vi "TestCMD.vi"(4 "QueueMotorCMD":refnum<queue>, 5 "ControlInterfce":variant, 6 "ID":string, 7 "MotorName":string) -> ()   [LabVIEW 2020]
panel:
  out "AddPath":T1(array[cluster])
  out "Speed":string
  out "Running?":bool=TRUE
  in  "CurrentPos":T2 {"X" format="%03.3f"; "Y" format="%3.3f"; "Z" format="%3.3f"; "U" format="%3.3f"; "V" format="%3.3f"; "W" format="%3.3f"; "H" format="%.3f"}
  out "CMD":T3
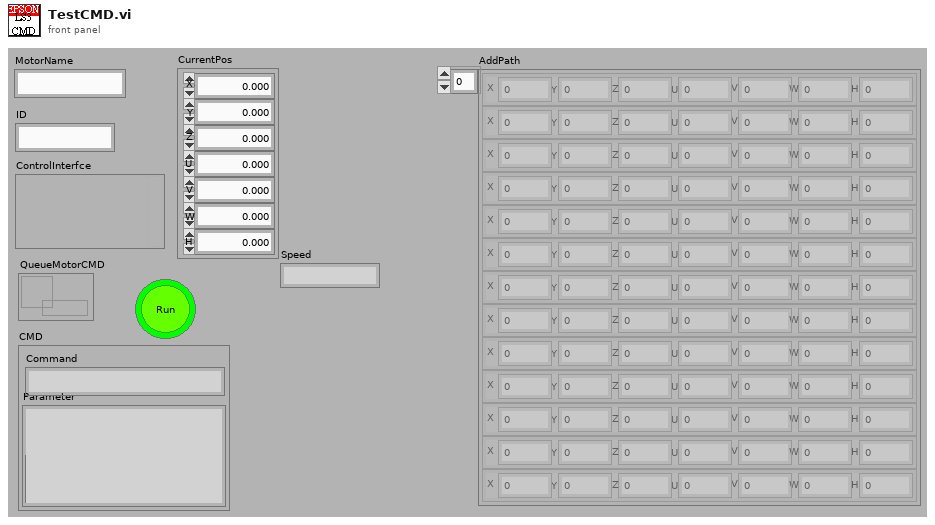
[diagram p1: front panel]
types:
  T1 = cluster{"X":sgl, "Y":sgl, "Z":sgl, "U":sgl, "V":sgl, "W":sgl, "H":sgl}[]
  T2 = cluster{"X":sgl, "Y":sgl, "Z":sgl, "U":sgl, "V":sgl, "W":sgl, "H":sgl}
  T3 = cluster{"Command":string, "Parameter":string, "queue out":refnum<queue>}
  T4 = enum16{"Get", "UpdatePointS", "Init", "UpdateIndex", "GetCurrent&Index+1", "GetWithIndex", "ChkLast"}
  T5 = enum16{"Get", "UpdatePointS", "Init", "UpdateIndex", "GetCurrent&Index+1", "GetWithIndex", "ChkLast", "GetCurrent"}
  T6 = cluster{cluster{"X":sgl, "Y":sgl, "Z":sgl, "U":sgl, "V":sgl, "W":sgl, "H":sgl}[]}
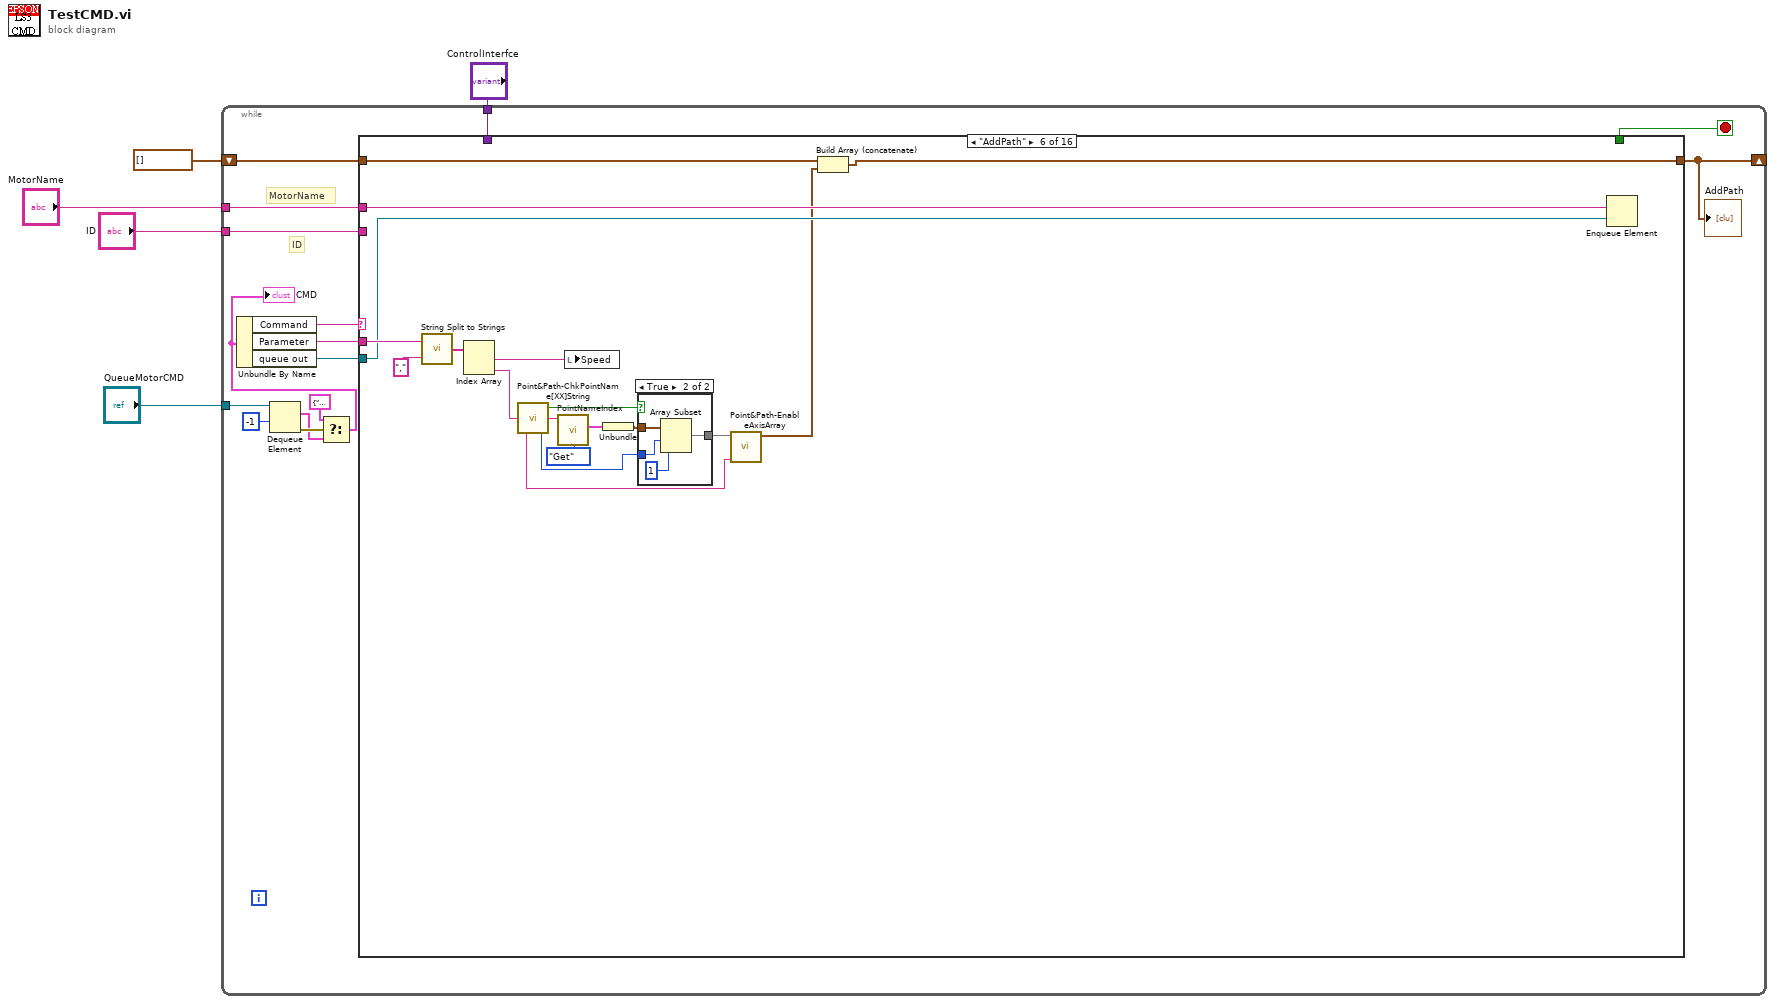
[diagram p0: block diagram]
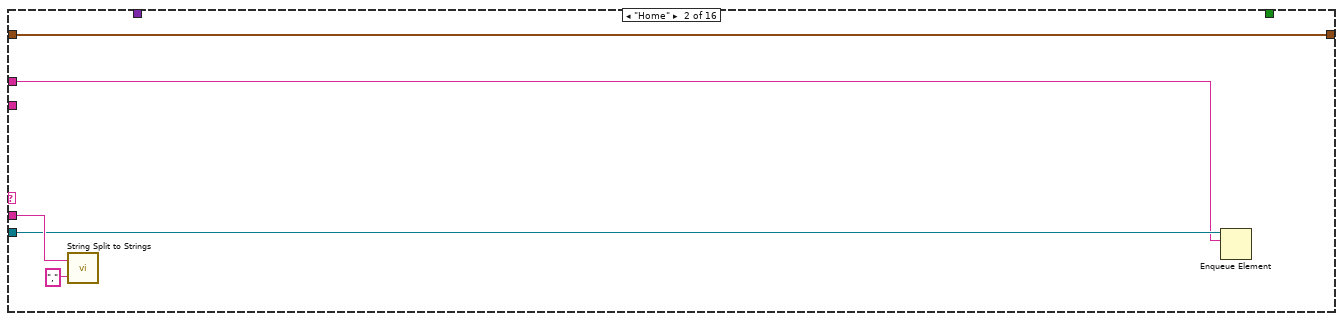
[diagram p3: hidden frame]
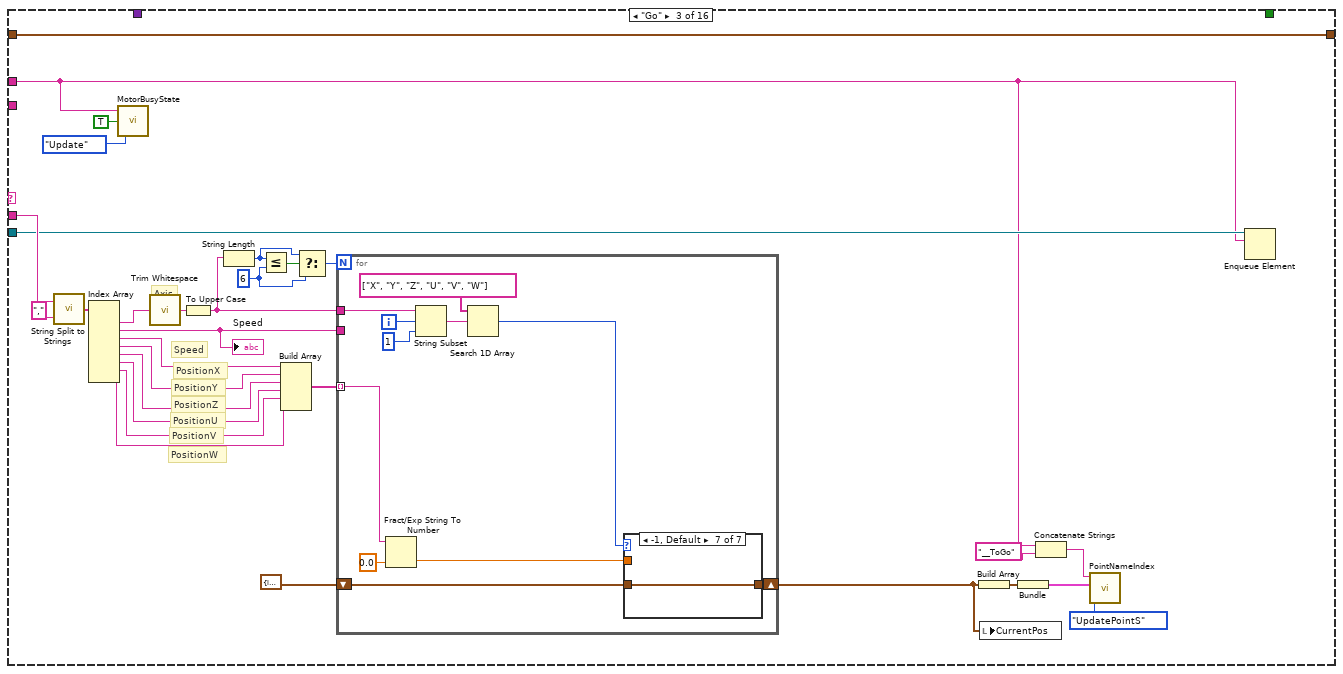
[diagram p4: hidden frame]
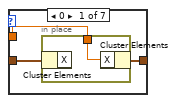
[diagram p5: hidden frame]
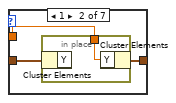
[diagram p6: hidden frame]
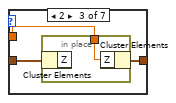
[diagram p7: hidden frame]
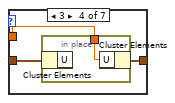
[diagram p8: hidden frame]
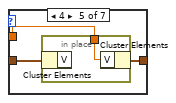
[diagram p9: hidden frame]
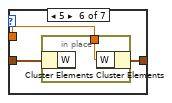
[diagram p10: hidden frame]
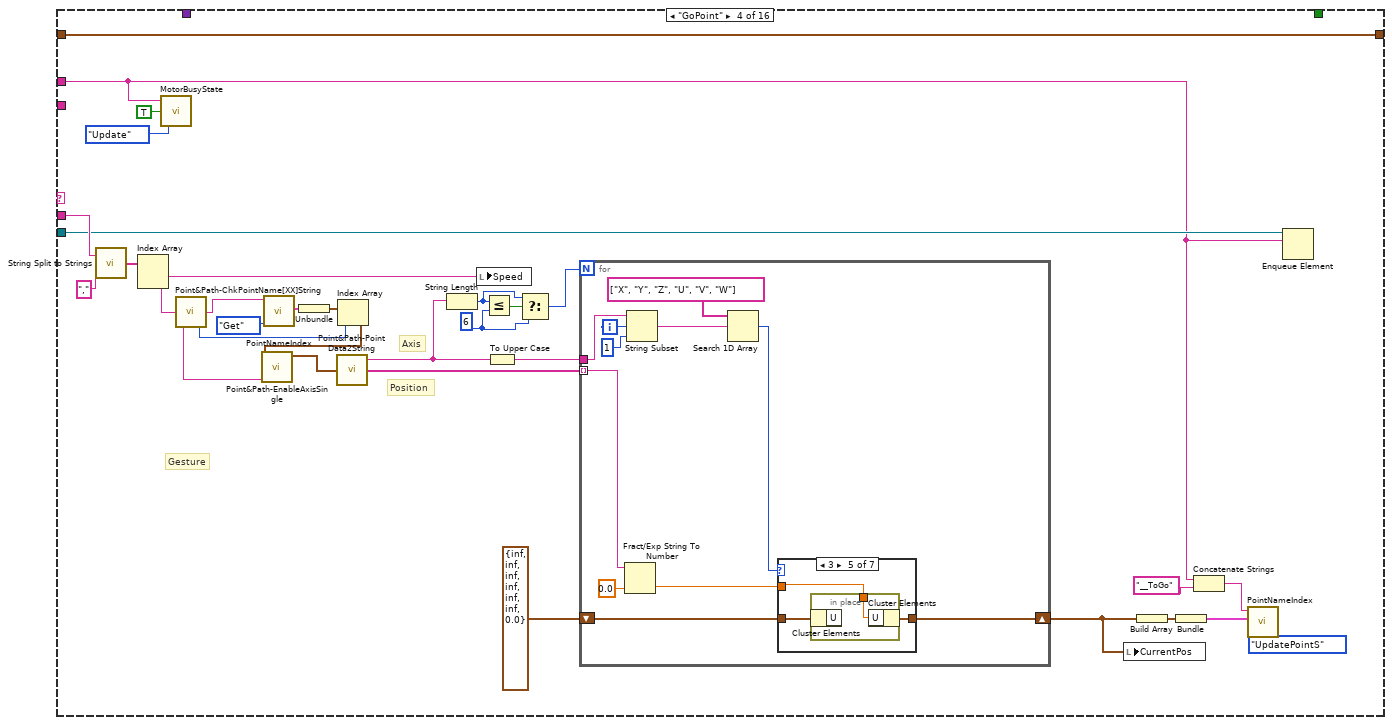
[diagram p11: hidden frame]
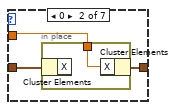
[diagram p13: hidden frame]
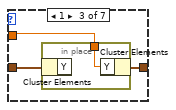
[diagram p14: hidden frame]
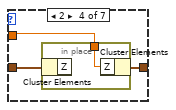
[diagram p15: hidden frame]
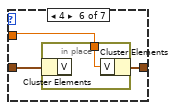
[diagram p16: hidden frame]
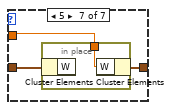
[diagram p17: hidden frame]
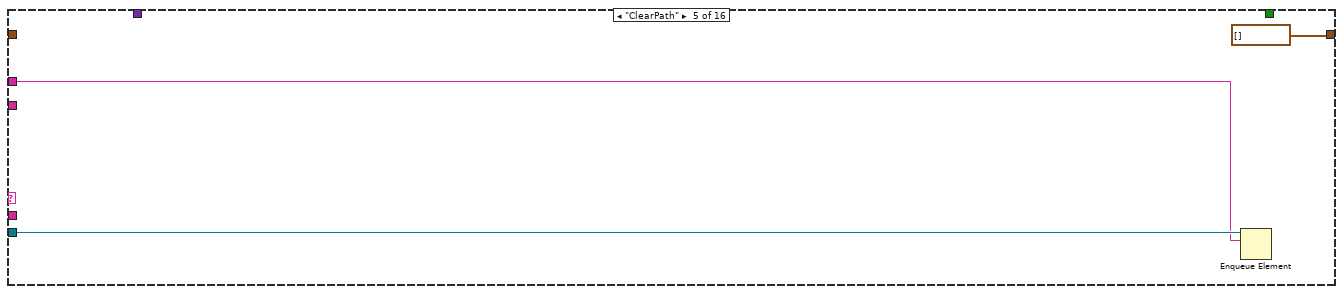
[diagram p18: hidden frame]
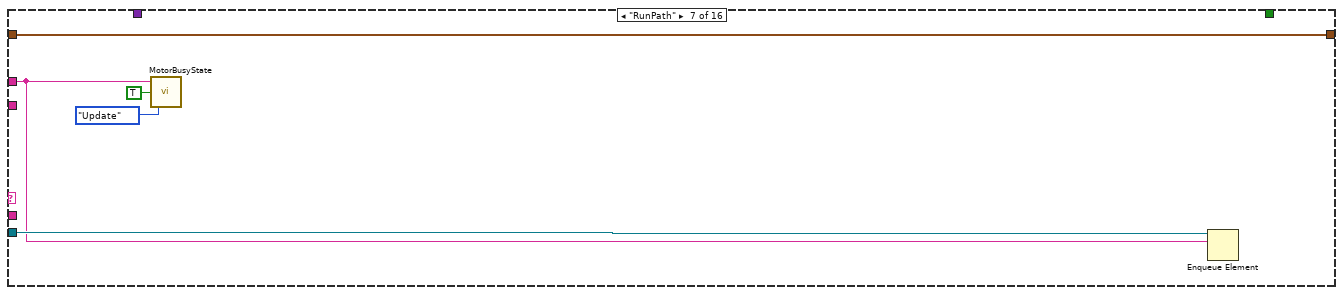
[diagram p20: hidden frame]
diagram:
  n1 = while {
    tunnel: "QueueMotorCMD" -> [w20]
    tunnel: "MotorName" -> [w16]
    tunnel: "ID" -> [w15]
    tunnel: "ControlInterfce" -> [w13]
    shift-right: [w6] -> _
    shift-left: T1 [] ("AddPath") -> [w7]
    stop <- w14 stop-if-true
    # "ID"
    # "MotorName"
    n2 = Dequeue Element(queue=w20, timeout in ms (-1)=-1) -> (element=w10:T3, error out=w11:errorcluster)  [unwired: 1 in, 2 out]
    n3 = Select(t=T3 {"Command"="Close", "Parameter"="", "queue out"=refnum} ("element"), s=w11, f=w10) -> (s? t:f=w9:T3)
    "CMD" <- w9
    n4 = Unbundle By Name(w9) -> ("Command"=w19:string, "Parameter"=w18:string, "queue out"=w17:refnum<queue>)
    n5 = case shown="\"AddPath\"" w19 {
      tunnel: w18 -> [_ w25 w48 w113 _ w176 _ _ _ _ _ _ _ _ _ _]
      tunnel: w17 -> [_ w24 w46 w106 w163 w170 w191 w194 w200 w205 w210 w214 _ w219 w223 _]
      tunnel: w16 -> [_ w23 w37 w99 w162 w174 w188 w193 w201 w207 w211 w213 _ _ _ _]
      tunnel: w15 -> [_ _ _ _ _ _ _ _ _ _ _ _ _ _ _ _]
      tunnel: [_ _ _ _ _ _ _ _ _ _ _ _ _ _ _ TRUE] -> w14
      tunnel: w13 -> [_ _ _ _ _ _ _ _ _ _ _ _ _ _ _ _]
      tunnel: w7 -> [w21 w22 w29 w93 _ w167 w187 w192 w195 w202 w209 w212 w215 w216 w220 w224]
      tunnel: [w21 w22 w29 w93 T1 [] ("AddPath") w166 w187 w192 w195 w202 w209 w212 w215 w216 w220 w224] -> w6
      frame "UpdateInfo", Default {
      }
      frame "Home" {
        n6 = call "String Split to Strings.vi"("search string/char (-)"=",", "String"=w25) -> ()  [unwired: 1 out]
        n7 = Enqueue Element(queue=w24, element=w23) -> ()  [unwired: 2 in, 3 out]
      }
      frame "Go" {
        w31 = 6 ("y")
        # "PositionW"
        # "PositionV"
        # "PositionU"
        # "PositionZ"
        # "PositionY"
        # "Speed"
        # "PositionX"
        # "Axis"
        n8 = call "String Split to Strings.vi"("search string/char (-)"=",", "String"=w48) -> ("Array"=w50:string[])
        n9 = Index Array(array=w50) -> (element #1=w51:string, element #2=w35:string, element #3=w52:string, element #4=w53:string, element #5=w54:string, element #6=w55:string, element #7=w28:string, element #8=w27:string)  [unwired: 8 in]
        "Speed" <- w35
        n10 = call "MotorBusyState.vi"("OP"=enum16{"Get", "Update", "Init"}."Update", "BusyStateIn"=TRUE, "MotorStateName"=w37) -> ()  [unwired: 1 in, 2 out]
        n11 = call <vilib>:"Trim Whitespace.vi"("string"=w51) -> ("trimmed string"=w56:string)  [unwired: 1 in]
        n12 = To Upper Case(1:w56) -> (0:w30:string)
        n13 = String Length(string=w30) -> (length=w33:i32)
        n14 = Less Or Equal?(x=w33, y=w31) -> (x <= y?=w34:bool)
        n15 = Build Array(w52, w53, w54, w55, w28, w27) -> (w47:string[])
        n16 = Select(t=w33, s=w34, f=w31) -> (s? t:f=w32:i32)
        n17 = for {
          N: w32 -> [_]
          tunnel: w30 -> [w64]
          tunnel: w47 -> [w61] mode=indexing
          shift-right: [w59] -> w36
          shift-left: T2 {"X"=inf, "Y"=inf, "Z"=inf, "U"=inf, "V"=inf, "W"=inf, "H"=0.0} ("PointData 2") -> [w62]
          tunnel: w35 -> [_]
          i -> [w65]
          n18 = Fract/Exp String To Number(string=w61, default (0 dbl)=sgl 0.0 ("default (0 DBL)")) -> (number=w57:sgl)  [unwired: 2 in, 1 out]
          n19 = String Subset(string=w64, offset (0)=w65, length (rest)=1 ("length (rest)")) -> (substring=w63:string)
          n20 = Search 1D Array(1D array=string[] ["X", "Y", "Z", "U", "V", "W"], element=w63) -> (index of element=w58:i32)  [unwired: 1 in]
          n21 = case shown="-1, Default" w58 {
            tunnel: w57 -> [w69 w73 w77 w81 w85 w89 _]
            tunnel: w62 -> [w70 w74 w78 w82 w86 w90 w92]
            tunnel: [w68 w72 w76 w80 w84 w88 w92] -> w59
            frame 0 {
              n22 = in-place {
                in-place-border: w69 -> [w71]
                n23 = in-place-cluster #1(w70) -> ()  [unwired: 1 out]
                n24 = in-place-cluster #1("X"=w71) -> (w68:T2)
              }
            }
            frame 1 {
              n25 = in-place {
                in-place-border: w73 -> [w75]
                n26 = in-place-cluster #2(w74) -> ()  [unwired: 1 out]
                n27 = in-place-cluster #2("Y"=w75) -> (w72:T2)
              }
            }
            frame 2 {
              n28 = in-place {
                in-place-border: w77 -> [w79]
                n29 = in-place-cluster #3(w78) -> ()  [unwired: 1 out]
                n30 = in-place-cluster #3("Z"=w79) -> (w76:T2)
              }
            }
            frame 3 {
              n31 = in-place {
                in-place-border: w81 -> [w83]
                n32 = in-place-cluster #4(w82) -> ()  [unwired: 1 out]
                n33 = in-place-cluster #4("U"=w83) -> (w80:T2)
              }
            }
            frame 4 {
              n34 = in-place {
                in-place-border: w85 -> [w87]
                n35 = in-place-cluster #5(w86) -> ()  [unwired: 1 out]
                n36 = in-place-cluster #5("V"=w87) -> (w84:T2)
              }
            }
            frame 5 {
              n37 = in-place {
                in-place-border: w89 -> [w91]
                n38 = in-place-cluster #6(w90) -> ()  [unwired: 1 out]
                n39 = in-place-cluster #6("W"=w91) -> (w88:T2)
              }
            }
            frame -1, Default {
            }
          }
        }
        n40 = Build Array(w36) -> (w43:T1)
        n41 = local write "CurrentPos"(w36) -> ()
        n42 = Bundle(w43) -> (w41:T6)  [unwired: 1 in]
        n43 = Concatenate Strings(w37, "__ToGo" ("string")) -> (w40:string)
        n44 = call "PointNameIndex.vi"("OP"=T4."UpdatePointS", "PointDataIn"=w41, "PointName"=w40) -> ()  [unwired: 3 in, 6 out]
        n45 = Enqueue Element(queue=w46, element=w37) -> ()  [unwired: 2 in, 3 out]
      }
      frame "GoPoint" {
        w108 = 6 ("y")
        # "Gesture"
        # "Position"
        # "Axis"
        n46 = call "String Split to Strings.vi"("search string/char (-)"=",", "String"=w113) -> ("Array"=w120:string[])
        n47 = Index Array(array=w120) -> (element #1=w94:string, element #2=w116:string)  [unwired: 2 in]
        n48 = call "MotorBusyState.vi"("OP"=enum16{"Get", "Update", "Init"}."Update", "BusyStateIn"=TRUE, "MotorStateName"=w99) -> ()  [unwired: 1 in, 2 out]
        n49 = call "Point&Path-ChkPointName[XX]String.vi"("PointName[XX]"=w116) -> ("Index"=w115:i32, "PointName"=w114:string, "EnableAxis"=w96:string)  [unwired: 1 in, 1 out]
        n50 = call "PointNameIndex.vi"("OP"=T4."Get", "PointName"=w114) -> ("PointDataOut"=w118:T6)  [unwired: 4 in, 5 out]
        n51 = Unbundle(w118) -> (w119:T1)
        n52 = Index Array(array=w119, index=w115) -> (element=w98:T2)
        n53 = call "Point&Path-EnableAxisSingle.vi"("PointDataIn"=w98, "EnableAxis"=w96) -> ("PointDataOut"=w97:T2)  [unwired: 8 in]
        n54 = call "Point&Path-PointData2String.vi"("Point"=w97) -> ("PositionStingArray"=w112:string[], "Axis"=w111:string)  [unwired: 2 in, 1 out]
        n55 = String Length(string=w111) -> (length=w109:i32)
        n56 = local write "Speed"(w94) -> ()
        n57 = Less Or Equal?(x=w109, y=w108) -> (x <= y?=w110:bool)
        n58 = To Upper Case(1:w111) -> (0:w124:string)
        n59 = Select(t=w109, s=w110, f=w108) -> (s? t:f=w107:i32)
        n60 = for {
          N: w107 -> [_]
          tunnel: w124 -> [w132]
          tunnel: w112 -> [w126] mode=indexing
          shift-right: [w128] -> w95
          shift-left: T2 {"X"=inf, "Y"=inf, "Z"=inf, "U"=inf, "V"=inf, "W"=inf, "H"=0.0} ("PointData 2") -> [w130]
          i -> [w133]
          n61 = Fract/Exp String To Number(string=w126, default (0 dbl)=sgl 0.0 ("default (0 DBL)")) -> (number=w125:sgl)  [unwired: 2 in, 1 out]
          n62 = String Subset(string=w132, offset (0)=w133, length (rest)=1 ("length (rest)")) -> (substring=w131:string)
          n63 = Search 1D Array(1D array=string[] ["X", "Y", "Z", "U", "V", "W"], element=w131) -> (index of element=w129:i32)  [unwired: 1 in]
          n64 = case shown="3" w129 {
            tunnel: w125 -> [_ w138 w142 w146 w150 w154 w158]
            tunnel: w130 -> [w136 w139 w143 w147 w151 w155 w159]
            tunnel: [w136 w137 w141 w145 w149 w153 w157] -> w128
            frame -1, Default {
            }
            frame 0 {
              n65 = in-place {
                in-place-border: w138 -> [w140]
                n66 = in-place-cluster #7(w139) -> ()  [unwired: 1 out]
                n67 = in-place-cluster #7("X"=w140) -> (w137:T2)
              }
            }
            frame 1 {
              n68 = in-place {
                in-place-border: w142 -> [w144]
                n69 = in-place-cluster #8(w143) -> ()  [unwired: 1 out]
                n70 = in-place-cluster #8("Y"=w144) -> (w141:T2)
              }
            }
            frame 2 {
              n71 = in-place {
                in-place-border: w146 -> [w148]
                n72 = in-place-cluster #9(w147) -> ()  [unwired: 1 out]
                n73 = in-place-cluster #9("Z"=w148) -> (w145:T2)
              }
            }
            frame 3 {
              n74 = in-place {
                in-place-border: w150 -> [w152]
                n75 = in-place-cluster #10(w151) -> ()  [unwired: 1 out]
                n76 = in-place-cluster #10("U"=w152) -> (w149:T2)
              }
            }
            frame 4 {
              n77 = in-place {
                in-place-border: w154 -> [w156]
                n78 = in-place-cluster #11(w155) -> ()  [unwired: 1 out]
                n79 = in-place-cluster #11("V"=w156) -> (w153:T2)
              }
            }
            frame 5 {
              n80 = in-place {
                in-place-border: w158 -> [w160]
                n81 = in-place-cluster #12(w159) -> ()  [unwired: 1 out]
                n82 = in-place-cluster #12("W"=w160) -> (w157:T2)
              }
            }
          }
        }
        n83 = local write "CurrentPos"(w95) -> ()
        n84 = Build Array(w95) -> (w103:T1)
        n85 = Bundle(w103) -> (w101:T6)  [unwired: 1 in]
        n86 = Concatenate Strings(w99, "__ToGo" ("string")) -> (w100:string)
        n87 = call "PointNameIndex.vi"("OP"=T4."UpdatePointS", "PointDataIn"=w101, "PointName"=w100) -> ()  [unwired: 3 in, 6 out]
        n88 = Enqueue Element(queue=w106, element=w99) -> ()  [unwired: 2 in, 3 out]
      }
      frame "ClearPath" {
        n89 = Enqueue Element(queue=w163, element=w162) -> ()  [unwired: 2 in, 3 out]
      }
      frame "AddPath" {
        n90 = call "String Split to Strings.vi"("search string/char (-)"=",", "String"=w176) -> ("Array"=w178:string[])
        n91 = Index Array(array=w178) -> (element #1=w164:string, element #2=w175:string)  [unwired: 2 in]
        n92 = call "Point&Path-ChkPointName[XX]String.vi"("PointName[XX]"=w175) -> ("Index"=w171:i32, "PointName"=w180:string, "Yes"=w173:bool, "EnableAxis"=w168:string)  [unwired: 1 in]
        n93 = call "PointNameIndex.vi"("OP"=T5."Get", "PointName"=w180) -> ("PointDataOut"=w181:T6)  [unwired: 4 in, 5 out]
        n94 = local write "Speed"(w164) -> ()
        n95 = Unbundle(w181) -> (w172:T1)
        n96 = case shown="True" w173 {
          tunnel: w172 -> [w182 w186]
          tunnel: [w182 w183] -> w169
          tunnel: w171 -> [_ w185]
          frame False {
          }
          frame True {
            n97 = Array Subset(array=w186, index=w185, length=1) -> (w183:T1)
          }
        }
        n98 = call "Point&Path-EnableAxisArray.vi"("PointDataIn"=w169, "EnableAxis"=w168) -> ("PointDataOut"=w165:T1)  [unwired: 8 in]
        n99 = Build Array (concatenate)(w167, w165) -> (w166:T1)
        n100 = Enqueue Element(queue=w170, element=w174) -> ()  [unwired: 2 in, 3 out]
      }
      frame "RunPath" {
        n101 = call "MotorBusyState.vi"("OP"=enum16{"Get", "Update", "Init"}."Update", "BusyStateIn"=TRUE, "MotorStateName"=w188) -> ()  [unwired: 1 in, 2 out]
        n102 = Enqueue Element(queue=w191, element=w188) -> ()  [unwired: 2 in, 3 out]
      }
      frame "Stop" {
        n103 = Enqueue Element(queue=w194, element=w193) -> ()  [unwired: 2 in, 3 out]
      }
      frame "GetPos" {
        # "Save to Point DataBase"
        n104 = Build Array("CurrentPos") -> (w199:T1)
        n105 = Bundle(w199) -> (w198:T6)  [unwired: 1 in]
        n106 = Enqueue Element(queue=w200, element=w201) -> ()  [unwired: 2 in, 3 out]
        n107 = call "PointNameIndex.vi"("OP"=T5."UpdatePointS", "PointDataIn"=w198, "PointName"=w201) -> ()  [unwired: 3 in, 6 out]
      }
      frame "GetState" {
        n108 = call "MotorBusyState.vi"("OP"=enum16{"Get", "Update", "Init"}."Update", "BusyStateIn"=FALSE, "MotorStateName"=w207) -> ("Busy?"=w204:bool)  [unwired: 1 in, 1 out]
        "Running?" <- w204
        n109 = To Variant(anything=w204) -> (Variant=w206:variant)
        n110 = Enqueue Element(queue=w205, element=w206) -> ()  [unwired: 2 in, 3 out]
      }
      frame "SetTool" {
        n111 = Enqueue Element(queue=w210, element=w211) -> ()  [unwired: 2 in, 3 out]
      }
      frame "ExtraCMD" {
        n112 = Enqueue Element(queue=w214, element=w213) -> ()  [unwired: 2 in, 3 out]
      }
      frame "SetDO" {
      }
      frame "GetDI" {
        n113 = To Variant(anything="") -> (Variant=w218:variant)
        n114 = Enqueue Element(queue=w219, element=w218) -> ()  [unwired: 2 in, 3 out]
      }
      frame "GetDO" {
        n115 = To Variant(anything="") -> (Variant=w222:variant)
        n116 = Enqueue Element(queue=w223, element=w222) -> ()  [unwired: 2 in, 3 out]
      }
      frame "Close" {
      }
    }
    "AddPath" <- w6
  }
